vi "popStack.vi"(8 "error in (no error)":errorcluster, 9 "pilha input":T1[](array[typedef]), 11 "Utilities in":refnum<class "Utilities.lvclass">) -> (0 "error out":errorcluster, 1 "pilha output":T1[](array[typedef]), 3 "Utilities out":refnum<class "Utilities.lvclass">)   [LabVIEW 2018, in "Utilities.lvclass"]
uses:
  Utilities.lvclass
  sslview/Util/segment.ctl
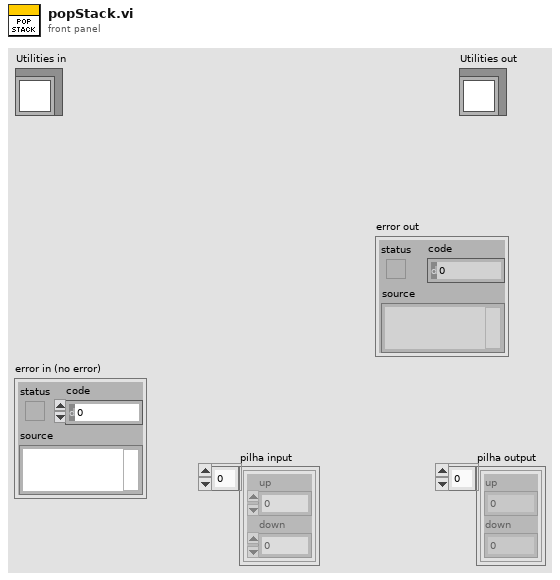
[diagram p1: front panel]
types:
  T1 = typedef "segment.ctl" = cluster{"up":dbl, "down":dbl}
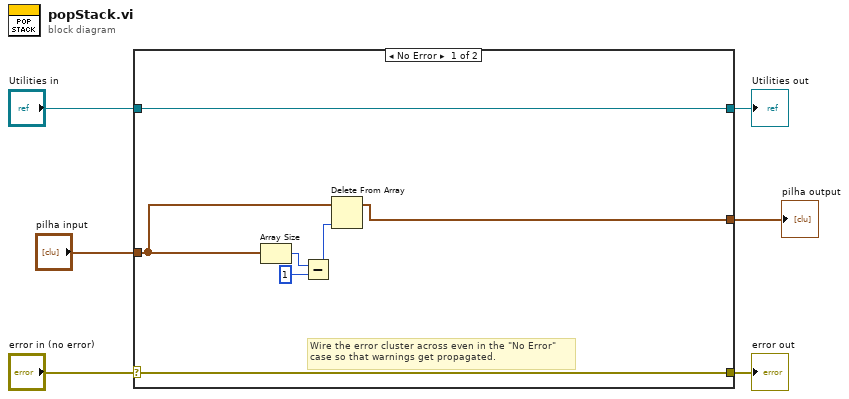
[diagram p0: block diagram]
diagram:
  n1 = case shown="No Error" "error in (no error)" {
    selector: "error in (no error)" -> [w12 w16]
    tunnel: [w12 w16] -> w5
    tunnel: [w13 w15] -> w3
    tunnel: "Utilities in" -> [w13 w15]
    tunnel: "pilha input" -> [w8 w14]
    tunnel: [w7 w14] -> w1
    frame No Error {
      # "Wire the error cluster across even in the \"No Error\"\ncase so that warnings get propagated."
      n2 = Array Size(array=w8) -> (size(s)=w11:i32)
      n3 = Subtract(x=w11, y=1) -> (x-y=w9:i32)
      n4 = Delete From Array(array=w8, index=w9) -> (array with subset deleted=w7:T1[])  [unwired: 1 in, 1 out]
    }
    frame Error {
    }
  }
  "error out" <- w5
  "Utilities out" <- w3
  "pilha output" <- w1
